vi "Result.Measurement Look Up Limits.vi"(0 "Meas":T1 {"Status" items=["LOG", "PASS", "FAIL", "ERROR"]}, 1 "error in":errorcluster, 4 "Limits":variant) -> (5 "Measurement Out":T1 {"Status" items=["LOG", "PASS", "FAIL", "ERROR"]})   [LabVIEW 2019]
uses:
  Result.Measurement Item.ctl
  Result.Measurement and Attribute Item Status.ctl
  Result.Test Limit Item.ctl
  Result.Limit Type.ctl
panel:
  in  "Test":bool
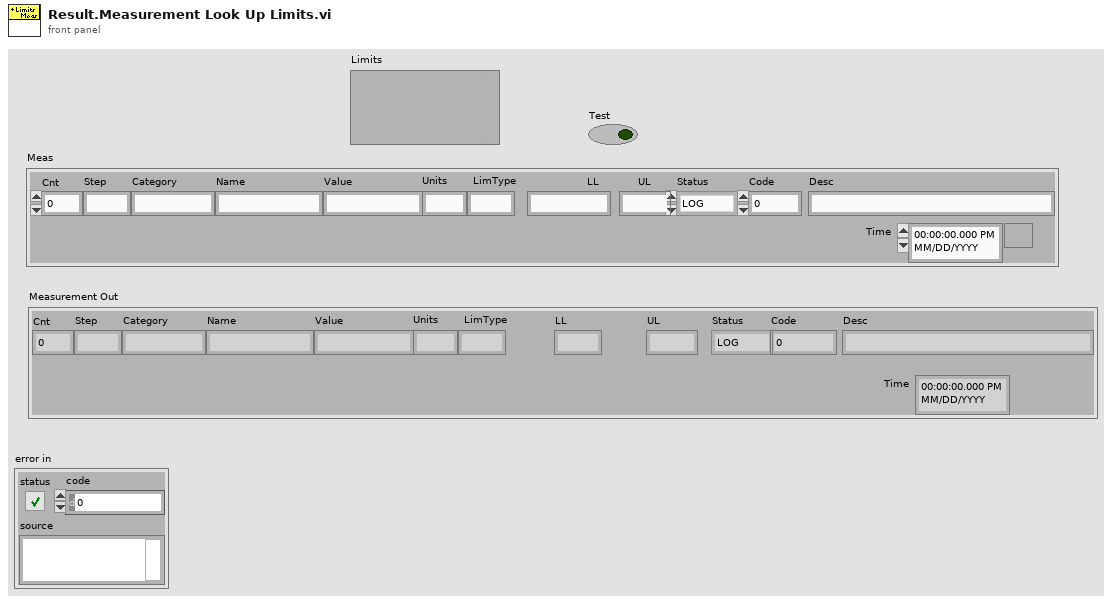
[diagram p1: front panel]
types:
  T1 = typedef "Result.Measurement Item.ctl" = cluster{"Cnt":i32, "Step":string, "Category":string, "Name":string, "Value":string, "Units":string, "LimType":string, "LL":string, "UL":string, "Status":T2, "Code":i32, "Desc":string, "Time":timestamp}
  T2 = typedef "Result.Measurement and Attribute Item Status.ctl" = i32
  T3 = typedef "Result.Test Limit Item.ctl" = cluster{"Name":string, "LimType":T4, "LL":string, "UL":string, "Units":string, "FailCode":i32, "FailDesc":string}
  T4 = typedef "Result.Limit Type.ctl" = enum16{"None", "EQ", "NE", "GT", "LT", "GE", "LE", "GTLT", "GELE", "GELT", "GTLE", "LTGT", "LEGE", "LEGT", "LTGE", "Contains", "NotContains"}
  T5 = enum16{"Time", "Error In", "Limits", "Fault Code", "Check Empty Code Desc", "Add Prefix", "Done"}
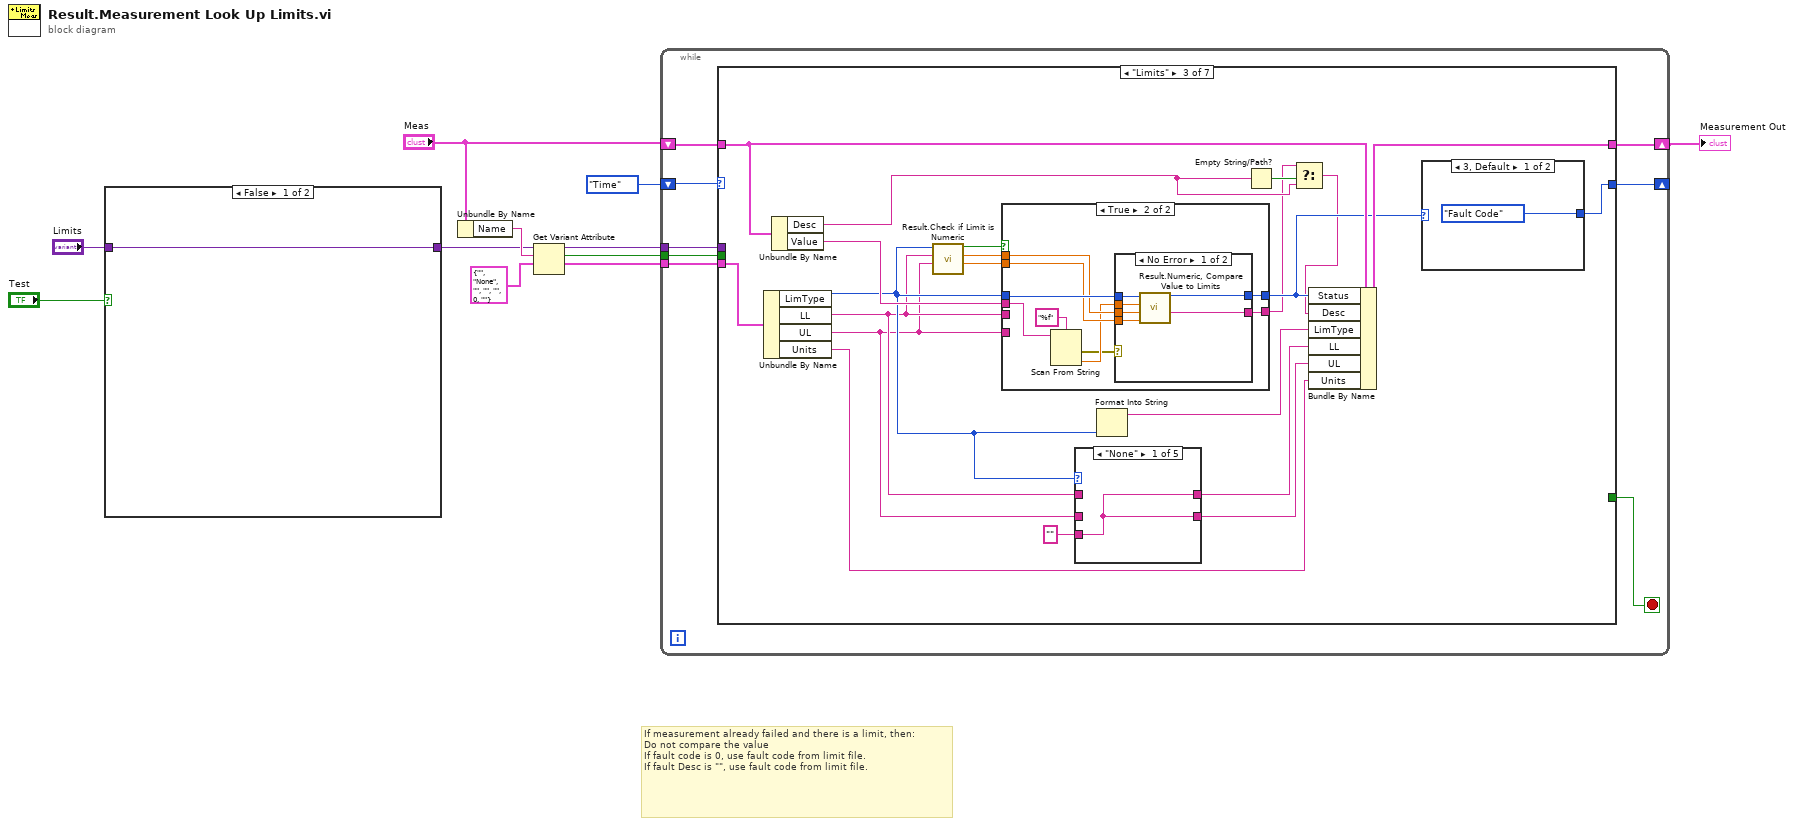
[diagram p0: block diagram]
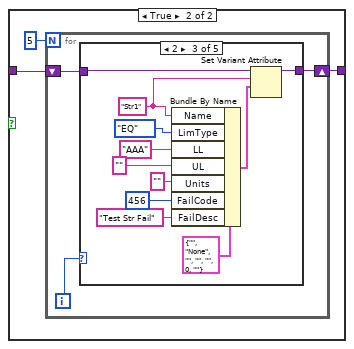
[diagram p2: hidden frame]
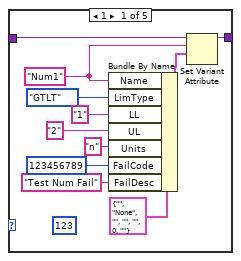
[diagram p3: hidden frame]
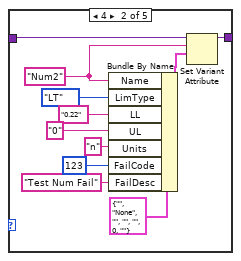
[diagram p4: hidden frame]
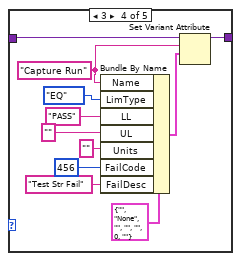
[diagram p5: hidden frame]
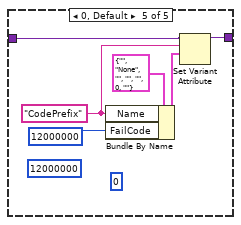
[diagram p6: hidden frame]
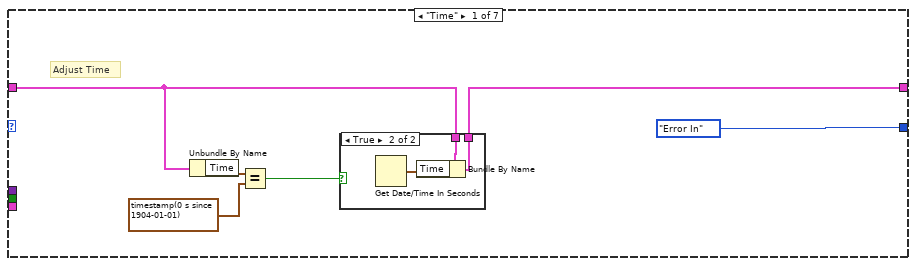
[diagram p7: hidden frame]
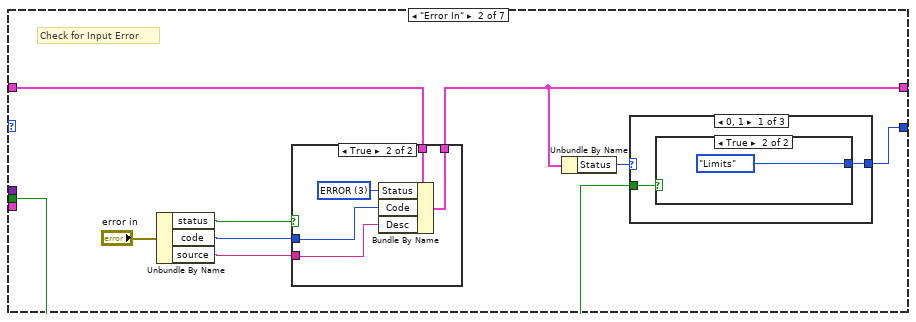
[diagram p9: hidden frame]
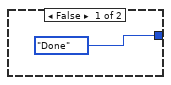
[diagram p10: hidden frame]
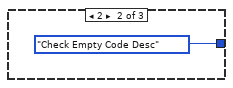
[diagram p11: hidden frame]
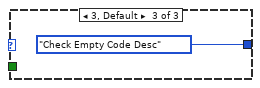
[diagram p12: hidden frame]
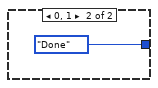
[diagram p18: hidden frame]
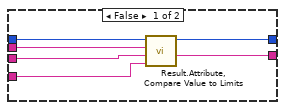
[diagram p19: hidden frame]
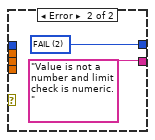
[diagram p20: hidden frame]
diagram:
  # "If measurement already failed and there is a limit, then:\nDo not compare the value\nIf fault code is 0, use fault code from limit file.\nIf fault Desc is \"\", use fault code from limit file."
  n1 = case shown="False" "Test" {
    tunnel: "Limits" -> [w12 w14]
    tunnel: [w12 w15] -> w4
    frame False {
    }
    frame True {
      n2 = for {
        N: 5 -> [_]
        shift-right: [w17] -> w15
        shift-left: w14 -> [w18]
        i -> [w16]
        n3 = case shown="2" w16 {
          tunnel: w18 -> [w21 w32 w41 w52 w64]
          tunnel: [w22 w33 w42 w53 w63] -> w17
          frame 1 {
            (unwired) 123 ("FailCode")
            w20 = "Num1" ("Name")
            n4 = Bundle By Name(cluster=T3 {"Name"="", "LimType"=enum."None", "LL"="", "UL"="", "Units"="", "FailCode"=0, "FailDesc"=""} ("Result.Test Limit Item"), "Name"=w20, "LimType"=Result.Limit_Type."GTLT", "LL"="1" ("Name"), "UL"="2" ("Name"), "Units"="n", "FailCode"=123456789, "FailDesc"="Test Num Fail") -> (w19:T3)
            n5 = Set Variant Attribute(Variant=w21, name=w20, value=w19) -> (Variant out=w22:variant)  [unwired: 1 in, 2 out]
          }
          frame 4 {
            w31 = "Num2" ("Name")
            n6 = Bundle By Name(cluster=T3 {"Name"="", "LimType"=enum."None", "LL"="", "UL"="", "Units"="", "FailCode"=0, "FailDesc"=""} ("Result.Test Limit Item"), "Name"=w31, "LimType"=Result.Limit_Type."LT", "LL"="0.22" ("Name"), "UL"="0" ("Name"), "Units"="n", "FailCode"=123, "FailDesc"="Test Num Fail") -> (w30:T3)
            n7 = Set Variant Attribute(Variant=w32, name=w31, value=w30) -> (Variant out=w33:variant)  [unwired: 1 in, 2 out]
          }
          frame 2 {
            w50 = "Str1" ("Name")
            n8 = Bundle By Name(cluster=T3 {"Name"="", "LimType"=enum."None", "LL"="", "UL"="", "Units"="", "FailCode"=0, "FailDesc"=""} ("Result.Test Limit Item"), "Name"=w50, "LimType"=Result.Limit_Type."EQ", "LL"="AAA" ("Name"), "UL"="" ("Name"), "Units"="", "FailCode"=456, "FailDesc"="Test Str Fail") -> (w51:T3)
            n9 = Set Variant Attribute(Variant=w41, name=w50, value=w51) -> (Variant out=w42:variant)  [unwired: 1 in, 2 out]
          }
          frame 3 {
            w61 = "Capture Run" ("Name")
            n10 = Bundle By Name(cluster=T3 {"Name"="", "LimType"=enum."None", "LL"="", "UL"="", "Units"="", "FailCode"=0, "FailDesc"=""} ("Result.Test Limit Item"), "Name"=w61, "LimType"=Result.Limit_Type."EQ", "LL"="PASS" ("Name"), "UL"="" ("Name"), "Units"="", "FailCode"=456, "FailDesc"="Test Str Fail") -> (w62:T3)
            n11 = Set Variant Attribute(Variant=w52, name=w61, value=w62) -> (Variant out=w53:variant)  [unwired: 1 in, 2 out]
          }
          frame 0, Default {
            (unwired) 0 ("FailCode")
            (unwired) 12000000 ("FailCode")
            w67 = "CodePrefix" ("Name")
            n12 = Bundle By Name(cluster=T3 {"Name"="", "LimType"=enum."None", "LL"="", "UL"="", "Units"="", "FailCode"=0, "FailDesc"=""} ("Result.Test Limit Item"), "Name"=w67, "FailCode"=12000000) -> (w68:T3)
            n13 = Set Variant Attribute(Variant=w64, name=w67, value=w68) -> (Variant out=w63:variant)  [unwired: 1 in, 2 out]
          }
        }
      }
    }
  }
  n14 = Unbundle By Name("Meas") -> ("Name"=w8:string)
  n15 = Get Variant Attribute(Variant=w4, name=w8, default value (empty Variant)=T3 {"Name"="", "LimType"=enum."None", "LL"="", "UL"="", "Units"="", "FailCode"=0, "FailDesc"=""} ("Result.Test Limit Item")) -> (duplicate Variant=w7:variant, found=w2:bool, value=w6:T3)  [unwired: 1 in, 1 out]
  n16 = while {
    shift-right: [w75] -> w3
    shift-left: "Meas" -> [w76]
    shift-right: [w72] -> _
    shift-left: T5."Time" -> [w73]
    tunnel: w7 -> [w71]
    tunnel: w6 -> [w70]
    tunnel: w2 -> [w69]
    stop <- w74 stop-if-true
    n17 = case shown="\"Limits\"" w73 {
      tunnel: w76 -> [w78 w91 w127 w165 w185 w209 w220]
      tunnel: [w79 w90 w126 w169 w186 w210 w220] -> w75
      tunnel: [_ _ _ _ _ _ TRUE] -> w74
      tunnel: [T5."Error In" w88 w123 T5."Check Empty Code Desc" T5."Add Prefix" T5."Done" T5."Done"] -> w72
      tunnel: w71 -> [_ _ _ _ _ w213 _]
      tunnel: w70 -> [_ _ w125 w170 w179 _ _]
      tunnel: w69 -> [_ w87 _ _ w177 _ _]
      frame "Time" {
        # "Adjust Time"
        n18 = Unbundle By Name(w78) -> ("Time"=w82:timestamp)
        n19 = Equal?(x=w82, y=timestamp(0 s since 1904-01-01)) -> (x = y?=w80:bool)
        n20 = case shown="True" w80 {
          tunnel: [w83 w85] -> w79
          tunnel: w78 -> [w83 w84]
          frame False {
          }
          frame True {
            n21 = Get Date/Time In Seconds() -> (seconds since 1Jan1904=w86:timestamp)
            n22 = Bundle By Name(cluster=w84, "Time"=w86) -> (w85:T1)
          }
        }
      }
      frame "Error In" {
        # "Check for Input Error"
        n23 = Unbundle By Name("error in") -> ("status"=w94:bool, "code"=w93:i32, "source"=w92:string)
        n24 = case shown="True" w94 {
          tunnel: w93 -> [_ w105]
          tunnel: w92 -> [_ w104]
          tunnel: w91 -> [w102 w107]
          tunnel: [w102 w103] -> w90
          frame False {
          }
          frame True {
            w106 = T2 3 items=["LOG", "PASS", "FAIL", "ERROR"] ("Status")
            n25 = Bundle By Name(cluster=w107, "Status"=w106, "Code"=w105, "Desc"=w104) -> (w103:T1)
          }
        }
        n26 = Unbundle By Name(w90) -> ("Status"=w89:T2)
        n27 = case shown="0, 1" w89 {
          tunnel: [w97 T5."Check Empty Code Desc" T5."Check Empty Code Desc"] -> w88
          tunnel: w87 -> [w96 _ _]
          frame 0, 1 {
            n28 = case shown="True" w96 {
              tunnel: [T5."Done" T5."Limits"] -> w97
              frame False {
              }
              frame True {
              }
            }
          }
          frame 2 {
          }
          frame 3, Default {
          }
        }
      }
      frame "Limits" {
        n29 = Unbundle By Name(w125) -> ("LimType"=w113:T4, "LL"=w112:string, "UL"=w111:string, "Units"=w118:string)
        n30 = Unbundle By Name(w127) -> ("Desc"=w116:string, "Value"=w128:string)
        n31 = call "Result.Check if Limit is Numeric.vi"("UL"=w111, "LL"=w112, "LimType"=w113) -> ("UL Num"=w108:dbl, "LL Num"=w109:dbl, "Is Numeric"=w110:bool)  [unwired: 6 in]
        n32 = case shown="True" w110 {
          tunnel: [w145 w154] -> w124
          tunnel: w113 -> [w144 w153]
          tunnel: w112 -> [w143 _]
          tunnel: w111 -> [w142 _]
          tunnel: [w141 w146] -> w115
          tunnel: w128 -> [w140 w151]
          tunnel: w109 -> [_ w150]
          tunnel: w108 -> [_ w149]
          frame False {
            n33 = call "Result.Attribute, Compare Value to Limits.vi"("UL"=w142, "LL"=w143, "Value"=w140, "LimType"=w144) -> ("Desc"=w141:string, "Status"=w145:T2)  [unwired: 6 in]
          }
          frame True {
            n34 = Scan From String(format string="%f", input string=w151) -> (error out=w147:errorcluster, output 1=w148:dbl)  [unwired: 3 in, 2 out]
            n35 = case shown="No Error" w147 {
              tunnel: [w160 w162] -> w154
              tunnel: w153 -> [w159 _]
              tunnel: w150 -> [w158 _]
              tunnel: w149 -> [w157 _]
              tunnel: w148 -> [w156 _]
              tunnel: [w155 "Value is not a number and limit check is numeric." ("Desc")] -> w146
              frame No Error {
                n36 = call "Result.Numeric, Compare Value to Limits.vi"("UL"=w157, "LL"=w158, "Value"=w156, "LimType"=w159) -> ("Desc"=w155:string, "Status"=w160:T2)  [unwired: 6 in]
              }
              frame Error {
                w162 = T2 2 items=["LOG", "PASS", "FAIL", "ERROR"] ("Status")
              }
            }
          }
        }
        n37 = case shown="\"None\"" w113 {
          tunnel: w112 -> [_ w131 w133 _ w136]
          tunnel: w111 -> [_ _ _ w134 w137]
          tunnel: "" -> [w129 w130 w132 w135 _]
          tunnel: [w129 w131 w133 w135 w136] -> w120
          tunnel: [w129 w130 w132 w134 w137] -> w119
          frame "None" {
          }
          frame "EQ".."GT", "GE" {
          }
          frame "Contains", "NotContains" {
          }
          frame "LT", "LE" {
          }
          frame Default {
          }
        }
        n38 = Format Into String(w113) -> (resulting string=w122:string)  [unwired: 3 in, 1 out]
        n39 = Empty String/Path?(string/path=w116) -> (empty?=w117:bool)
        n40 = Select(t=w115, s=w117, f=w116) -> (s? t:f=w114:string)
        n41 = Bundle By Name(cluster=w127, "Status"=w124, "Desc"=w114, "LimType"=w122, "LL"=w120, "UL"=w119, "Units"=w118) -> (w126:T1)
        n42 = case shown="3, Default" w124 {
          tunnel: [T5."Fault Code" T5."Done"] -> w123
          frame 3, Default {
          }
          frame 0, 1 {
          }
        }
      }
      frame "Fault Code" {
        # "Keep existing description if oen is provided"
        n43 = Unbundle By Name(w165) -> ("Desc"=w164:string)
        n44 = Unbundle By Name(w170) -> ("FailCode"=w167:i32, "FailDesc"=w173:string)
        n45 = Empty String/Path?(string/path=w164) -> (empty?=w172:bool)
        n46 = Less Than 0?(x=w167) -> (x < 0?=w168:bool)
        n47 = case shown="True" w168 {
          tunnel: [w174 w175] -> w166
          frame False {
            w174 = T2 2 items=["LOG", "PASS", "FAIL", "ERROR"] ("Status")
          }
          frame True {
            w175 = T2 3 items=["LOG", "PASS", "FAIL", "ERROR"] ("Status")
          }
        }
        n48 = Select(t=w173, s=w172, f=w164) -> (s? t:f=w171:string)
        n49 = Bundle By Name(cluster=w165, "Status"=w166, "Code"=w167, "Desc"=w171) -> (w169:T1)
      }
      frame "Check Empty Code Desc" {
        n50 = Unbundle By Name(w179) -> ("FailCode"=w178:i32, "FailDesc"=w176:string)
        n51 = Unbundle By Name(w185) -> ("Status"=w183:T2, "Code"=w184:i32)
        n52 = case shown="0" w184 {
          tunnel: w185 -> [w195 w201]
          tunnel: w183 -> [_ w199]
          tunnel: [w195 w198] -> w182
          tunnel: w177 -> [_ w197]
          tunnel: w178 -> [_ w196]
          frame Default {
          }
          frame 0 {
            n53 = case shown="False" w197 {
              tunnel: [w203 w206] -> w200
              tunnel: w199 -> [w202 _]
              tunnel: w196 -> [_ w206]
              frame False {
                n54 = case shown="3, Default" w202 {
                  tunnel: [-5000 ("Code") 5000 ("Code")] -> w203
                  frame 3, Default {
                  }
                  frame 2 {
                  }
                }
              }
              frame True {
              }
            }
            n55 = Bundle By Name(cluster=w201, "Code"=w200) -> (w198:T1)
          }
        }
        n56 = Unbundle By Name(w182) -> ("Desc"=w181:string)
        n57 = case shown="\"\"" w181 {
          tunnel: w182 -> [w187 w192]
          tunnel: [w187 w191] -> w186
          tunnel: w177 -> [_ w189]
          tunnel: w176 -> [_ w188]
          frame Default {
          }
          frame "" {
            n58 = case shown="False" w189 {
              tunnel: ["No description assigned to this failure." ("Desc") w194] -> w190
              tunnel: w188 -> [_ w194]
              frame False {
              }
              frame True {
              }
            }
            n59 = Bundle By Name(cluster=w192, "Desc"=w190) -> (w191:T1)
          }
        }
      }
      frame "Add Prefix" {
        n60 = Get Variant Attribute(Variant=w213, name="CodePrefix", default value (empty Variant)=T3 {"Name"="", "LimType"=enum."None", "LL"="", "UL"="", "Units"="", "FailCode"=0, "FailDesc"=""} ("Result.Test Limit Item")) -> (value=w215:T3)  [unwired: 1 in, 3 out]
        n61 = Unbundle By Name(w215) -> ("FailCode"=w212:i32)
        n62 = Unbundle By Name(w209) -> ("Code"=w208:i32)
        n63 = Less Than 0?(x=w208) -> (x < 0?=w207:bool)
        n64 = call "TestExec.Append Fault Code Prefix_V2.vi"("Positive(F)\\Negative(T)"=w207, "FaultCode"=w208, "FaultCode Prefix"=w212) -> ("New Fault Code"=w211:i32)  [unwired: 8 in]
        n65 = Bundle By Name(cluster=w209, "Code"=w211) -> (w210:T1)
      }
      frame "Done", Default {
      }
    }
  }
  "Measurement Out" <- w3
